vi "SimpleMotorFeedForward_Example.vi"() -> ()   [LabVIEW 2019]
uses:
  <vilib>/Rock Robotics/WPI/ThirdParty/JAS_Junk/TrajLib/LinearFilter_ResetToValue.vi
  <vilib>/Rock Robotics/WPI/ThirdParty/JAS_Junk/TrajLib/LinearFilter_Calculate.vi
  <vilib>/Rock Robotics/WPI/ThirdParty/JAS_Junk/TrajLib/SimpleMotorFF_Calculate.vi
  <vilib>/Rock Robotics/WPI/ThirdParty/JAS_Junk/TrajLib/VI/TimeInterpDouble_CleanUp.vi
  <vilib>/Rock Robotics/WPI/ThirdParty/JAS_Junk/TrajLib/MathUtil_Interpolate.vi
  <vilib>/Rock Robotics/WPI/ThirdParty/JAS_Junk/TrajLib/MathUtil_Clamp.vi
  <vilib>/Rock Robotics/WPI/ThirdParty/JAS_Junk/TrajLib/LinearFilter_MovingAverage.vi
  <vilib>/Rock Robotics/WPI/ThirdParty/JAS_Junk/TrajLib/LinearFilter_LowPassBW1.vi
  <vilib>/Rock Robotics/WPI/ThirdParty/JAS_Junk/TrajLib/LinearFilter_LowPassBW2.vi
  <vilib>/Rock Robotics/WPI/ThirdParty/JAS_Junk/TrajLib/LinearFilter_HighPassBW1.vi
  <vilib>/Rock Robotics/WPI/ThirdParty/JAS_Junk/TrajLib/LinearFilter_HighPassBW2.vi
  <vilib>/gmath/interp.llb/Search Ordered Table.vi
  <vilib>/Rock Robotics/WPI/ThirdParty/JAS_Junk/TrajLib/Trajectory_Library.lvlib
panel:
  out "Rate":dbl
  in  "Tab Control":T1(tab)
  out "Sampling On":bool
  in  "Ka Helper Sampling On/Off":bool
  out "Filtered Setpoint \nRate of Change":dbl format="%11.3f"
  in  "Auto Setpoint":bool
  out "CO Trend":dbl(graph)
  out "SP, PV Trend":T2(graph)
  in  "Desired Speed":dbl(slide)=-0.22222222222222499 scale=-10.0..10.0 scale format="%#.1f"
  in  "Enable Noise":bool
  in  "Ks":dbl format="%#_13g"
  in  "Kv":dbl=0.1 format="%#_13g"
  in  "Ka":dbl format="%#_13g"
  out "Motor Dmd":dbl format="%13.3f"
  out "Filtered Speed":dbl format="%12.2f"
  out "Filtered Speed \nError":dbl format="%11.3f"
  in  "Speed Setpoint\n to find":dbl=4.0 format="%#_13g"
  out "Ka":dbl
  out "SP Found":bool
  in  "Calc Ka":bool
  out "PV Found":bool
  out "SP time":dbl format="%#_15g"
  out "PV time":dbl format="%#_15g"
  out "SP Verify":dbl
  out "Co verify":dbl
  # "Simple Motor Feedforward Example"
  # "FT/SEC"
  # "FT/SEC"
  # "Sample procedure to tune Simple Motor Feedforward Ks, Kv, Ka.\n\nThis is just one possible method to do the tuning.  Other methods, including using the characterization tool, can be used.\n\n1) Set the Ka and Ks to 0.0.   Set Kv to be 1 / Estimated Maximum Speed.   (For many robots 10 feet/sec works as a starting point).\n     If using any closed loop control, such as a PID, disable the closed loop control, either by removing the code, or for the advanced\n    PID, putting it in manual mode.  (This simulation does not have a closed loop controller.)\n\n2)  Set the motor output at a small value.  (Example 0.15).  To do this set the speed demand to a small value, such as 1.5 Ft/Sec.\n      After the robot comes to constant speed, record the Motor Demand CO and Actual Speed (PV)\n\n3) Set the motor output to a large value (Example 0.90).   To do this, set the speed demand to a large value, such as 9.0 Ft/Sec\n     After the robot (or this simulation) comes to a constant speed, record the Motor Demand (CO) and the Actual Speed (PV).\n\n4) Ks and Kv can be calculated from the straight line equation:\n                               Motor Dmd CO = Sign( Speed_Setpoint) x Ks + Speed_Setpoint x Kv\n                                          Sign = 1 when Speed_Setoint > 0.0, \n                                          0 when Speed_Setpoint = 0 and, \n                                          -1 when Speed_Setpoint < 0\n\n5) The Ka term represents the additional Motor Demand CO needed to cancel the lag of the motor.   Technically, the Ka term\n      represents a \"lead\" function (sometimes referred to as a kicker circuit).  The amount that Ka adds to the Motor Demand CO\n      is  Ka x Speed_Setpoint Rate of Change (units/second).  Therefore, while the speed is ramping, one knows, or can be\n      calculated:   \n                             - Setpoint Rate of Change\n                             - Speed, speed setpoint, motor demand a time \"n\"\n                             - motor demand at time \"m\" where speed_m = speed_setpoint_n\n  \n    This should be enough data to calculate a value for Ka:\n                              Ka = (motor_demand_m - motor_demand_n ) / setpoint_rate_of_change\n\n     The Ka term will cause the speed to overshoot slightly during a ramp.  This is an expected side-affect of this type of \n     algorithm.  \n\n6) Test everything and look at the trend to ensure the response is acceptable.    Adjust as desired."
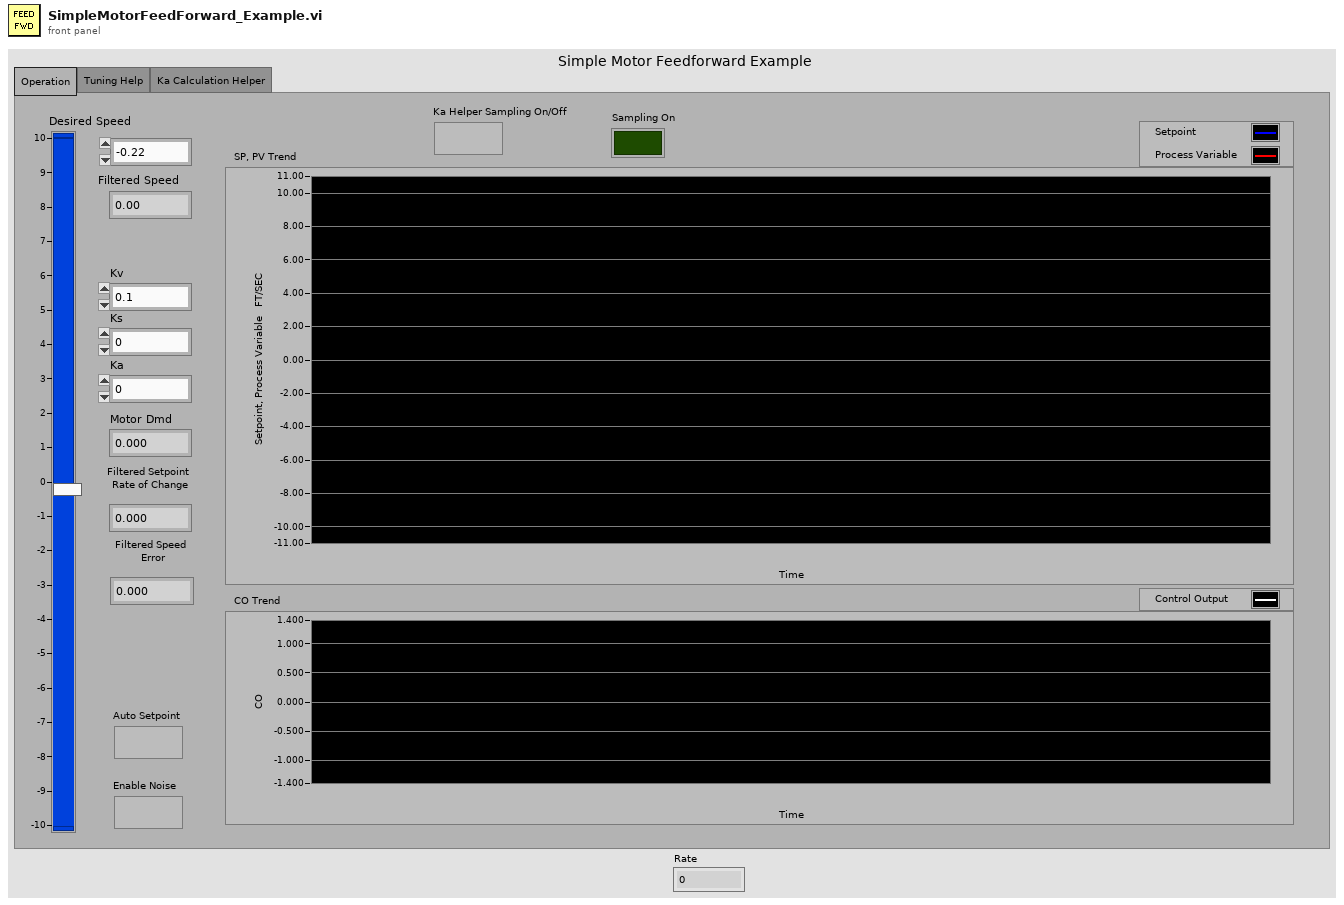
[diagram p1: front panel]
types:
  T1 = enum32{"Operation", "Tuning Help", "Ka Calculation Helper"}
  T2 = cluster{"SpeedSetpoint":dbl, "LeftWheelSpeed":dbl}
  T3 = typedef "Trajectory_Library.lvlib/TIME_INTERPOLATABLE_DOUBLE.ctl" = cluster{"TimeStamps":dbl[], "DoubleValue":dbl[], "Min_TimeStamp":dbl, "Max_TimeStamp":dbl, "ItemCount":i32, "MaxBufferTime":dbl}
  T4 = enum16{"Moving Average", "Low Pass 1st Order Butterworth", "Low Pass 2nd Order Butterworth", "High Pass 1st Order Butterworth", "High Pass 2nd Order Butterworth"}
  T5 = typedef "Trajectory_Library.lvlib/SIMPLE_MOTOR_FF.ctl" = cluster{"Ks":dbl, "Kv":dbl, "Ka":dbl, "KnInv":dbl}
  T6 = cluster{"Speed Setpoint Ft/Sec":dbl, "Motor Speed":dbl}
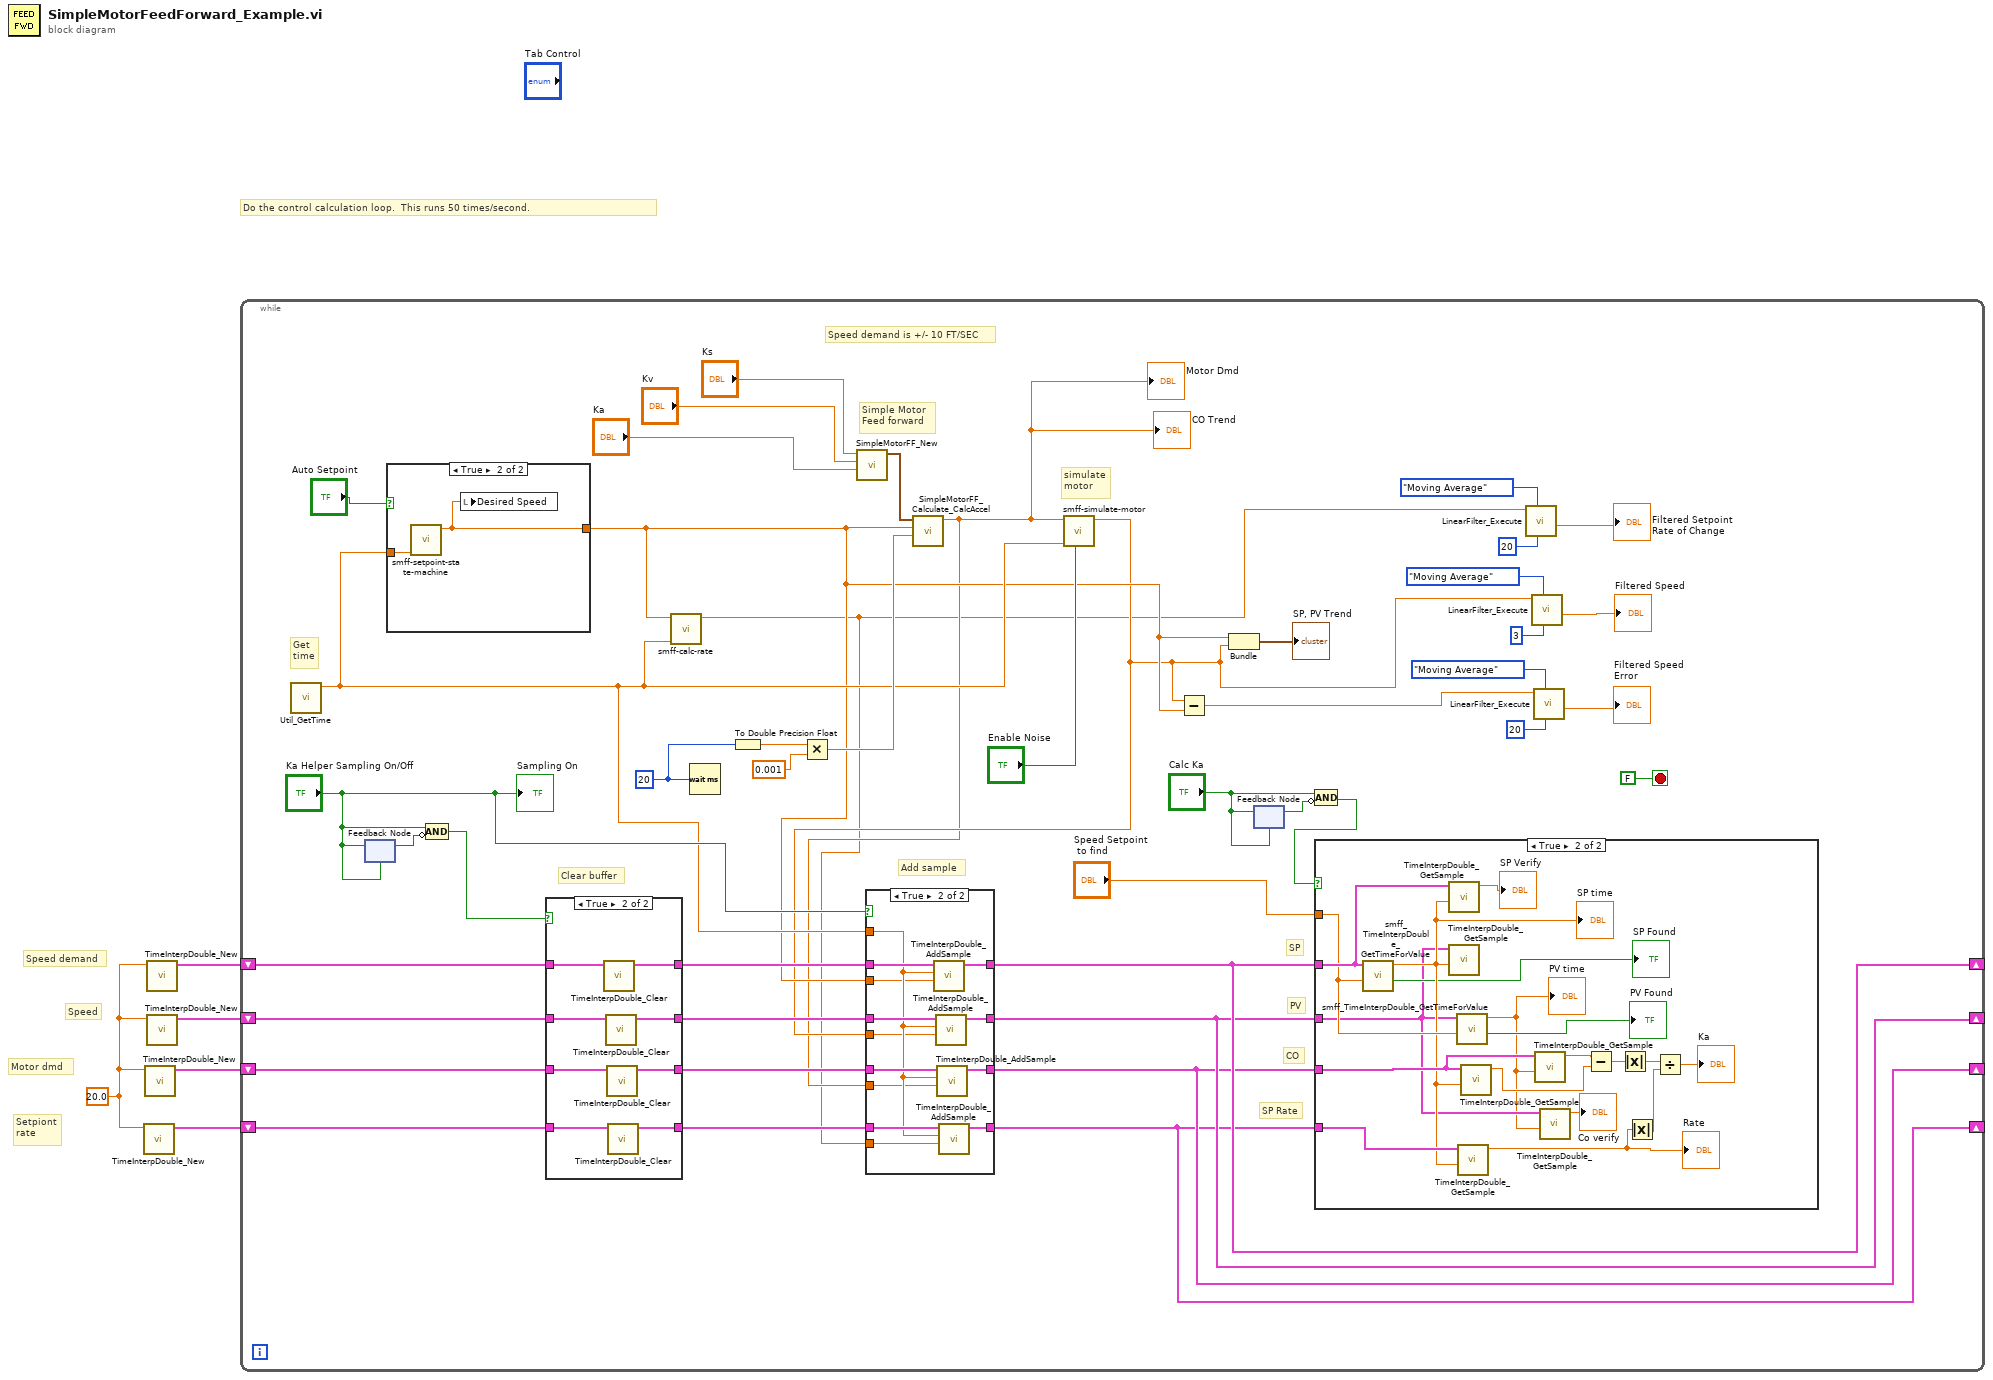
[diagram p0: block diagram]
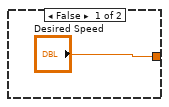
[diagram p5: hidden frame]
diagram:
  w5 = 20.0 ("MaxTime")
  # "Setpiont\nrate"
  # "Motor dmd"
  # "Speed"
  # "Speed demand"
  # "Do the control calculation loop.  This runs 50 times/second."
  n1 = call <vilib>:"TimeInterpDouble_New.vi"("MaxTime"=w5) -> ("TimeInterpDouble"=w4:T3)  [unwired: 10 in]
  n2 = call <vilib>:"TimeInterpDouble_New.vi"("MaxTime"=w5) -> ("TimeInterpDouble"=w3:T3)  [unwired: 10 in]
  n3 = call <vilib>:"TimeInterpDouble_New.vi"("MaxTime"=w5) -> ("TimeInterpDouble"=w1:T3)  [unwired: 10 in]
  n4 = call <vilib>:"TimeInterpDouble_New.vi"("MaxTime"=w5) -> ("TimeInterpDouble"=w2:T3)  [unwired: 10 in]
  n5 = while {
    shift-right: [w9] -> _
    shift-left: w1 -> [w27]
    shift-right: [w8] -> _
    shift-left: w2 -> [w26]
    shift-right: [w7] -> _
    shift-left: w3 -> [w25]
    shift-right: [w6] -> _
    shift-left: w4 -> [w24]
    stop <- FALSE stop-if-true
    w50 = u32 20 ("milliseconds to wait")
    # "SP Rate"
    # "SP"
    # "CO"
    # "PV"
    # "Add sample"
    # "Clear buffer"
    # "Get\ntime"
    # "Speed demand is +/- 10 FT/SEC"
    # "simulate\nmotor"
    # "Simple Motor\nFeed forward"
    n6 = call <vilib>:"Util_GetTime.vi"() -> ("FPGA_Time_Seconds"=w22:dbl)  [unwired: 10 in, 1 out]
    n7 = feedback-in #1("Ka Helper Sampling On/Off") -> ()
    n8 = feedback #1("Ka Helper Sampling On/Off") -> (w29:bool)
    n9 = case shown="True" "Auto Setpoint" {
      tunnel: w22 -> [_ w101]
      tunnel: ["Desired Speed" w100] -> w17
      frame False {
      }
      frame True {
        n10 = call "smff-setpoint-state-machine.vi"("Time pass through"=w101) -> ("Speed Setpoint Ft/Sec"=w100:dbl)  [unwired: 9 in, 1 out]
        n11 = local write "Desired Speed"(w100) -> ()
      }
    }
    n12 = Compound Arithmetic op=AND("Ka Helper Sampling On/Off", invert w29) -> (w28:bool)
    n13 = case shown="True" w28 {
      tunnel: w27 -> [w90 w98]
      tunnel: w26 -> [w89 w97]
      tunnel: w25 -> [w88 w96]
      tunnel: w24 -> [w87 w95]
      tunnel: [w90 w94] -> w21
      tunnel: [w89 w93] -> w20
      tunnel: [w88 w92] -> w19
      tunnel: [w87 w91] -> w18
      frame False {
      }
      frame True {
        n14 = call <vilib>:"TimeInterpDouble_Clear.vi"("in TimeInterpDouble"=w98) -> ("out TimeInterpDouble"=w94:T3)  [unwired: 10 in]
        n15 = call <vilib>:"TimeInterpDouble_Clear.vi"("in TimeInterpDouble"=w97) -> ("out TimeInterpDouble"=w93:T3)  [unwired: 10 in]
        n16 = call <vilib>:"TimeInterpDouble_Clear.vi"("in TimeInterpDouble"=w96) -> ("out TimeInterpDouble"=w92:T3)  [unwired: 10 in]
        n17 = call <vilib>:"TimeInterpDouble_Clear.vi"("in TimeInterpDouble"=w95) -> ("out TimeInterpDouble"=w91:T3)  [unwired: 10 in]
      }
    }
    n18 = call "smff-calc-rate.vi"("Time pass through"=w22, "Value"=w17) -> ("Value Rate"=w14:dbl)  [unwired: 9 in]
    n19 = Wait (ms)(milliseconds to wait=w50) -> ()  [unwired: 1 out]
    n20 = To Double Precision Float(number=w50) -> (double precision float=w44:dbl)
    n21 = Multiply(x=w44, y=0.001) -> (x*y=w42:dbl)
    n22 = call <vilib>:"SimpleMotorFF_New.vi"("Ka"="Ka", "Kv"="Kv", "Ks"="Ks") -> ("SIMPLE_MOTOR_FF"=w48:T5)  [unwired: 8 in]
    n23 = call <vilib>:"SimpleMotorFF_Calculate_CalcAccel.vi"("dT_Sec"=w42, "VelSp"=w17, "SIMPLE_MOTOR_FF"=w48) -> ("FeedForward"=w15:dbl)  [unwired: 8 in]
    "Motor Dmd" <- w15
    "CO Trend" <- w15
    n24 = call "smff-simulate-motor.vi"("Use Noise"="Enable Noise", "Time"=w22, "CO-ControlOutput"=w15) -> ("Motor Speed"=w16:dbl)  [unwired: 8 in]
    n25 = case shown="True" "Ka Helper Sampling On/Off" {
      tunnel: w22 -> [_ w82]
      tunnel: w21 -> [w73 w86]
      tunnel: w20 -> [w72 w85]
      tunnel: w19 -> [w71 w84]
      tunnel: w18 -> [w70 w83]
      tunnel: w17 -> [_ w81]
      tunnel: w16 -> [_ w80]
      tunnel: w15 -> [_ w79]
      tunnel: w14 -> [_ w78]
      tunnel: [w73 w77] -> w9
      tunnel: [w72 w76] -> w8
      tunnel: [w70 w75] -> w6
      tunnel: [w71 w74] -> w7
      frame False {
      }
      frame True {
        n26 = call <vilib>:"TimeInterpDouble_AddSample.vi"("Value"=w81, "TimeStamp"=w82, "in TimeInterpDouble"=w86) -> ("out TimeInterpDouble"=w77:T3)  [unwired: 7 in, 1 out]
        n27 = call <vilib>:"TimeInterpDouble_AddSample.vi"("Value"=w80, "TimeStamp"=w82, "in TimeInterpDouble"=w85) -> ("out TimeInterpDouble"=w76:T3)  [unwired: 7 in, 1 out]
        n28 = call <vilib>:"TimeInterpDouble_AddSample.vi"("Value"=w79, "TimeStamp"=w82, "in TimeInterpDouble"=w84) -> ("out TimeInterpDouble"=w74:T3)  [unwired: 7 in, 1 out]
        n29 = call <vilib>:"TimeInterpDouble_AddSample.vi"("Value"=w78, "TimeStamp"=w82, "in TimeInterpDouble"=w83) -> ("out TimeInterpDouble"=w75:T3)  [unwired: 7 in, 1 out]
      }
    }
    n30 = Subtract(x=w16, y=w17) -> (x-y=w40:dbl)
    n31 = Bundle("Speed Setpoint Ft/Sec"=w17, "Motor Speed"=w16) -> (→"SP, PV Trend":T6)  [unwired: 1 in]
    n32 = feedback #2("Calc Ka") -> (w13:bool)
    n33 = feedback-in #2("Calc Ka") -> ()
    n34 = Compound Arithmetic op=AND("Calc Ka", invert w13) -> (w11:bool)
    n35 = case shown="True" w11 {
      tunnel: "Speed Setpoint\n to find" -> [_ w67]
      tunnel: w9 -> [_ w68]
      tunnel: w8 -> [_ w56]
      tunnel: w6 -> [_ w69]
      tunnel: w7 -> [_ w66]
      frame False {
      }
      frame True {
        n36 = call "smff_TimeInterpDouble_GetTimeForValue.vi"("ValueToFind"=w67, "TimeInterpDouble"=w68) -> ("ValueFound"=→"SP Found":bool, "TimeStamp"=w65:dbl)  [unwired: 8 in]
        "SP time" <- w65
        n37 = call <vilib>:"TimeInterpDouble_GetSample.vi"("TimeStamp"=w65, "TimeInterpDouble"=w68) -> ("OutputDouble"=→"SP Verify":dbl)  [unwired: 8 in, 1 out]
        n38 = call <vilib>:"TimeInterpDouble_GetSample.vi"("TimeStamp"=w65, "TimeInterpDouble"=w56) -> ()  [unwired: 8 in, 2 out]
        n39 = call "smff_TimeInterpDouble_GetTimeForValue.vi"("ValueToFind"=w67, "TimeInterpDouble"=w56) -> ("ValueFound"=→"PV Found":bool, "TimeStamp"=w55:dbl)  [unwired: 8 in]
        "PV time" <- w55
        n40 = call <vilib>:"TimeInterpDouble_GetSample.vi"("TimeStamp"=w65, "TimeInterpDouble"=w69) -> ("OutputDouble"=w52:dbl)  [unwired: 8 in, 1 out]
        "Rate" <- w52
        n41 = call <vilib>:"TimeInterpDouble_GetSample.vi"("TimeStamp"=w65, "TimeInterpDouble"=w66) -> ("OutputDouble"=w63:dbl)  [unwired: 8 in, 1 out]
        n42 = call <vilib>:"TimeInterpDouble_GetSample.vi"("TimeStamp"=w55, "TimeInterpDouble"=w66) -> ("OutputDouble"=w64:dbl)  [unwired: 8 in, 1 out]
        n43 = call <vilib>:"TimeInterpDouble_GetSample.vi"("TimeStamp"=w55, "TimeInterpDouble"=w56) -> ("OutputDouble"=→"Co verify":dbl)  [unwired: 8 in, 1 out]
        n44 = Subtract(x=w64, y=w63) -> (x-y=w62:dbl)
        n45 = Absolute Value(x=w62) -> (abs(x)=w61:dbl)
        n46 = Absolute Value(x=w52) -> (abs(x)=w53:dbl)
        n47 = Divide(x=w61, y=w53) -> (x/y=→"Ka":dbl)
      }
    }
    n48 = call <vilib>:"LinearFilter_Execute.vi"("Samples"=20, "Filter Type"=T4."Moving Average", "Input"=w14) -> ("Output"=→"Filtered Setpoint \nRate of Change":dbl)  [unwired: 7 in, 1 out]
    n49 = call <vilib>:"LinearFilter_Execute.vi"("Samples"=3, "Filter Type"=T4."Moving Average", "Input"=w16) -> ("Output"=→"Filtered Speed":dbl)  [unwired: 7 in, 1 out]
    n50 = call <vilib>:"LinearFilter_Execute.vi"("Samples"=20, "Filter Type"=T4."Moving Average", "Input"=w40) -> ("Output"=→"Filtered Speed \nError":dbl)  [unwired: 7 in, 1 out]
    "Sampling On" <- "Ka Helper Sampling On/Off"
  }
